vi "add_node_object_dictionary.vi"(8 "type":u16, 9 "subind":u8, 10 "index":u16, 11 "node":u8) -> (3 "return":i16)   [LabVIEW 2011]
uses:
  canopen_dll_master.dll
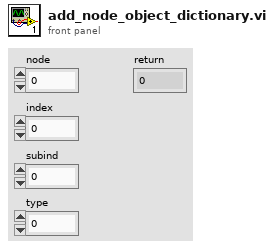
[diagram p1: front panel]
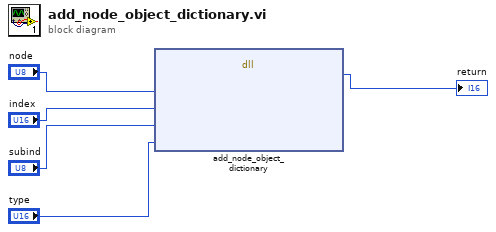
[diagram p0: block diagram]
diagram:
  n1 = dll-call lib="canopen_dll_master.dll" fn="add_node_object_dictionary"("node"="node", "index"="index", "subind"="subind", "type"="type") -> ("return type"=→"return":i16)  [unwired: 7 in, 2 out]
